vi "DS BaseActor Polling Interval.vi"() -> ()   [LabVIEW 2015, in "CS++Utilities.lvlib"]
doc: "Activate or deactivate CS++PVProxy when using DataSocket."
uses:
  CS++Utilities.lvlib
panel:
  in  "Pollin Interval URL":string="dstp://localhost/CSPP_Core_SV/myBaseActor_PollingInterval"
  in  "Polling Interval?":dbl[unit]=10.0
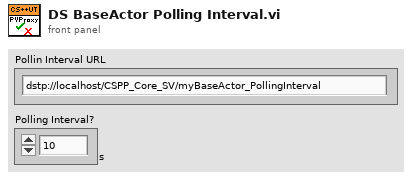
[diagram p1: front panel]
types:
  T1 = enum16{"Read", "Write", "ReadWrite", "BufferedRead", "BufferedReadWrite"}
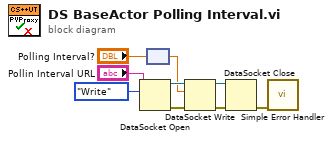
[diagram p0: block diagram]
diagram:
  n1 = DataSocket Open(10:T1."Write" ("mode"), 11:"Pollin Interval URL") -> (0:w8:errorcluster, 3:w6:refnum<k13>)  [unwired: 2 in]
  n2 = node("Polling Interval?") -> (w1:dbl)
  n3 = DataSocket Write(8:w8, 10:w1, 11:w6) -> (0:w4:errorcluster, 3:w3:refnum<k13>)  [unwired: 1 in, 1 out]
  n4 = DataSocket Close(8:w4, 11:w3) -> (0:w2:errorcluster)  [unwired: 1 in, 1 out]
  n5 = call <vilib>:"Simple Error Handler.vi"("error in (no error)"=w2) -> ()  [unwired: 4 in, 5 out]
